vi "DFT_exapmle.vi"() -> ()   [LabVIEW 2018]
doc: "dft exapmle: This example is an example of discrete Fourier transform, which is a commonly used frequency domain analysis technique used to convert time-domain signals or images into the frequency domain for spectral analysis, filtering, compression, and other operations."
uses:
  vi.lib/VIRobotics/opencv_yiku/Mat/Mat_8U/Mat_8U.lvclass
  C:/Program Files/National Instruments/LabVIEW 2018/vi.lib/VIRobotics/opencv_yiku/Mat/Mat/Mat.lvclass
  vi.lib/VIRobotics/opencv_yiku/Mat/Mat_32F/Mat_32F.lvclass
  vi.lib/VIRobotics/opencv_yiku/Mat/Create_Mat_32F.vi
  vi.lib/VIRobotics/opencv_yiku/Cap/Cap.lvclass
  vi.lib/VIRobotics/opencv_yiku/opencv_yiku.lvlib
  vi.lib/VIRobotics/opencv_yiku/Mat/Mat/Mat.lvclass
panel:
  in  "stop":bool
  out "idft":sgl[][](graph)
  out "im":sgl[][](graph)
  out "re":sgl[][](graph)
  out "new picture":picture
  # "1.Make sure your computer has a camera."
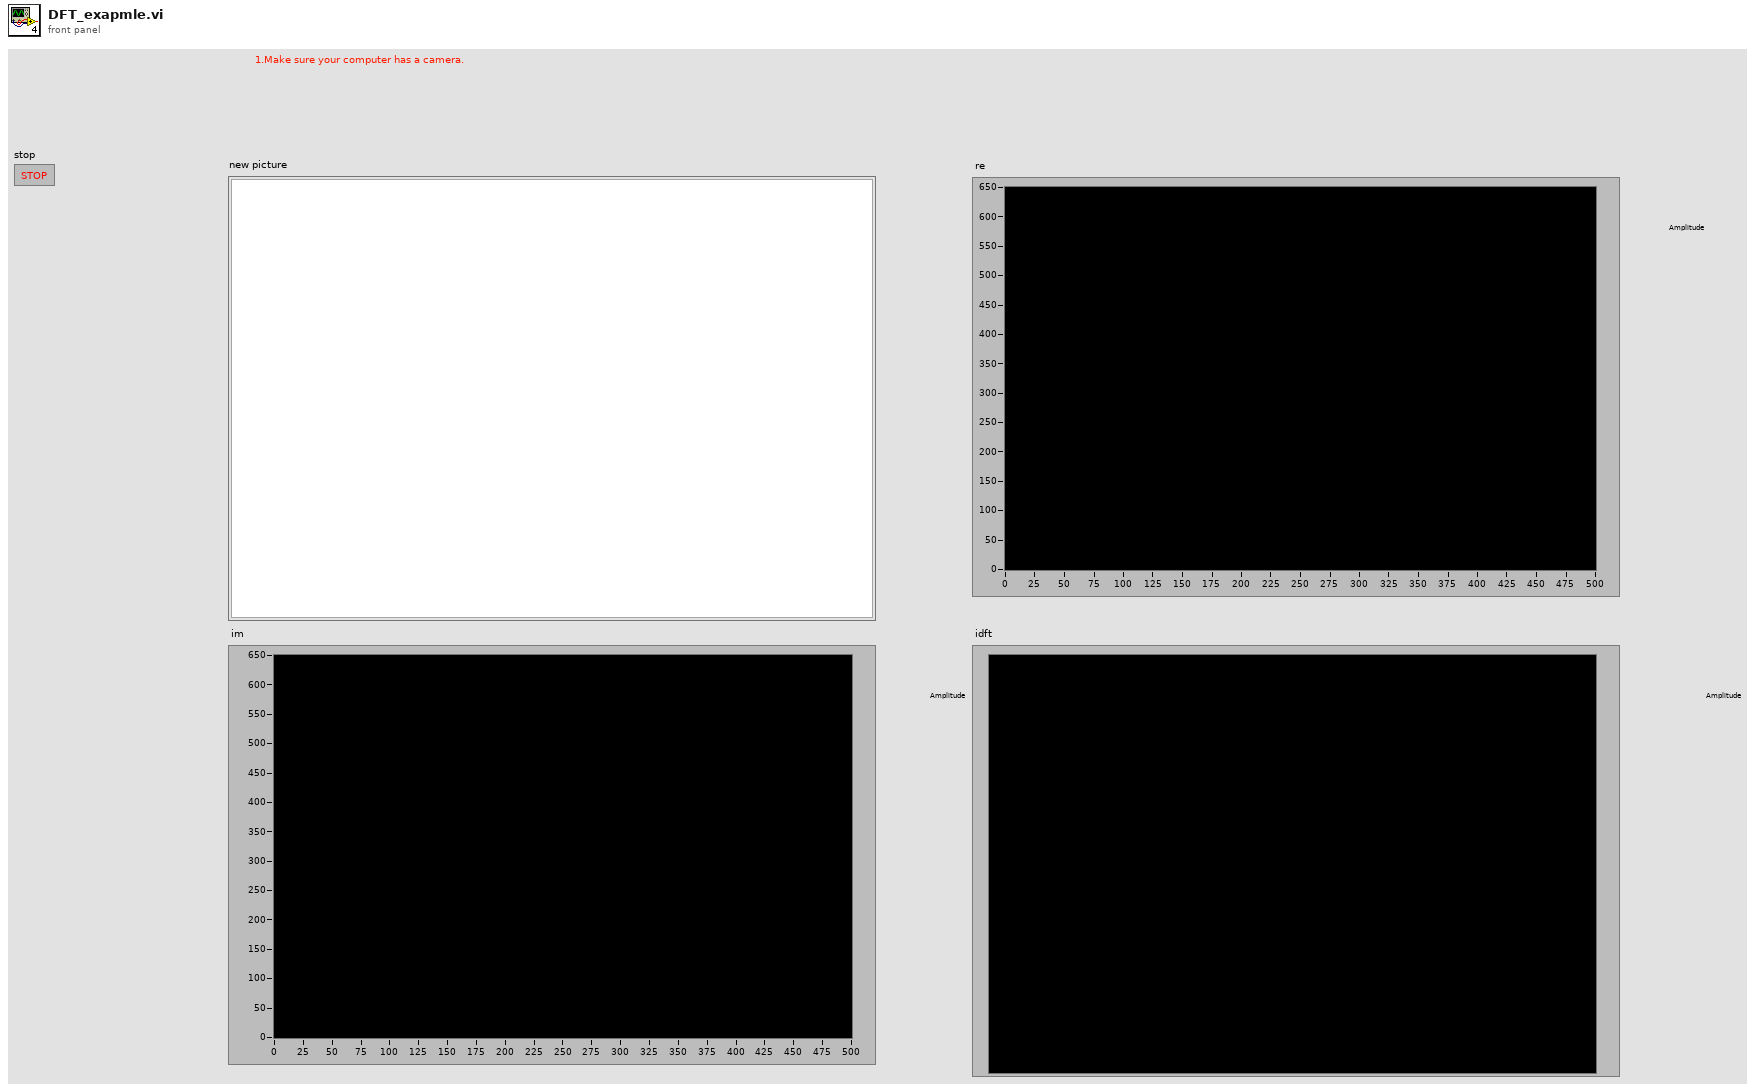
[diagram p1: front panel]
types:
  T1 = enum16{"COLOR_BGR2BGRA", "COLOR_BGRA2BGR", "COLOR_BGR2RGBA", "COLOR_RGBA2BGR", "COLOR_BGR2RGB", "COLOR_BGRA2RGBA", "COLOR_BGR2GRAY", "COLOR_RGB2GRAY", "COLOR_GRAY2BGR", "COLOR_GRAY2BGRA"}
  T2 = typedef "imagedata.ctl" = cluster{"image type":i32, "image depth":i32, "image":u8[], "mask":u8[], "colors":u32[], "Rectangle":cluster{"left":i16, "top":i16, "right":i16, "bottom":i16}}
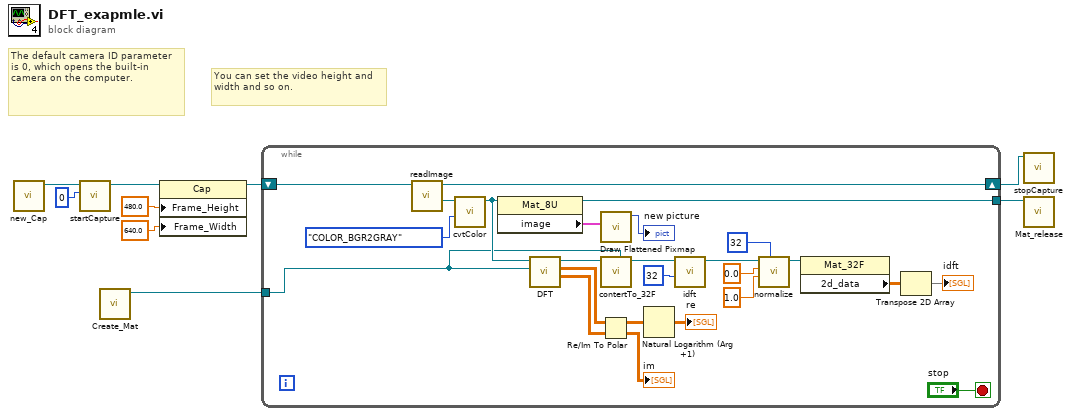
[diagram p0: block diagram]
diagram:
  # "You can set the video height and width and so on."
  # "The default camera ID parameter is 0, which opens the built-in camera on the computer."
  n1 = call "new_Cap.vi"() -> ("Cap out"=w9:refnum<class "Cap.lvclass">)  [unwired: 10 in, 1 out]
  n2 = call "startCapture.vi"("cameraID"=0, "Cap in"=w9) -> ("Cap out"=w6:refnum<class "Cap.lvclass">)  [unwired: 8 in, 1 out]
  n3 = call-poly "Create_Mat.vi"() -> ("Mat_32F_out"=w1:refnum<class "Mat_32F.lvclass">)  [unwired: 10 in, 1 out]
  n4 = property class="Cap"(reference=w6, "Frame_Height"=480.0, "Frame_Width"=640.0) -> (reference out=w5:refnum<class "Cap.lvclass">)  [unwired: 1 in, 1 out]
  n5 = while {
    shift-right: [w34] -> w7
    shift-left: w5 -> [w32]
    tunnel: w1 -> [w10]
    tunnel: [w31] -> w2
    stop <- "stop" stop-if-true
    n6 = call "readImage.vi"("Cap in"=w32) -> ("Mat out"=w33:refnum<class "Mat_8U.lvclass">, "Cap out"=w34:refnum<class "Cap.lvclass">)  [unwired: 8 in, 1 out]
    n7 = call "cvtColor.vi"("dstCn"=T1."COLOR_BGR2GRAY", "src"=w33) -> ("src out"=w30:refnum<class "Mat_8U.lvclass">)  [unwired: 7 in, 2 out]
    n8 = property class="Mat_8U"(reference=w30) -> (reference out=w31:refnum<class "Mat_8U.lvclass">, "image"=w26:T2)  [unwired: 1 in, 1 out]
    n9 = call "DFT.vi"("Mat_32F"=w10, "Mat"=w30) -> ("Im"=w27:sgl[][], "Re"=w28:sgl[][], "Mat_32F out"=w13:refnum<class "Mat_32F.lvclass">)  [unwired: 6 in, 1 out]
    n10 = call <vilib>:"Draw Flattened Pixmap.vi"("image data"=w26) -> ("new picture"=→"new picture":picture)  [unwired: 8 in]
    n11 = call "contertTo_32F.vi"("dst in"=w10, "Mat"=w13) -> ("dst out"=w12:refnum<class "Mat_32F.lvclass">)  [unwired: 9 in]
    n12 = Re/Im To Polar(2:w27, 3:w28) -> (0:→"im":sgl[][], 1:w22:sgl[][])
    n13 = Natural Logarithm (Arg +1)(1:w22) -> (0:→"re":sgl[][])
    n14 = call "idft.vi"("flags"=32, "src"=w12) -> ("dst"=w14:refnum<class "Mat_32F.lvclass">)  [unwired: 8 in, 1 out]
    n15 = call "normalize.vi"("norm_type"=32, "beta"=1.0, "alpha"=0.0, "Mat"=w14) -> ("Mat_out"=w29:refnum<class "Mat_32F.lvclass">)  [unwired: 6 in, 1 out]
    n16 = property class="Mat_32F"(reference=w29) -> ("2d_data"=w24:sgl[][])  [unwired: 1 in, 2 out]
    n17 = Transpose 2D Array(2D array=w24) -> (transposed array=→"idft":sgl[][])
  }
  n18 = call "stopCapture.vi"("Cap in"=w7) -> ()  [unwired: 10 in, 1 out]
  n19 = call "Mat_release.vi"("Mat in"=w2) -> ()  [unwired: 10 in, 1 out]
